vi "Read Ship States.vi"(11 "TCP Refnum In":refnum<k5>) -> (2 "Eta_ship":dbl[](array[numeric]), 3 "TCP Refnum Out":refnum<k5>)   [LabVIEW 2014]
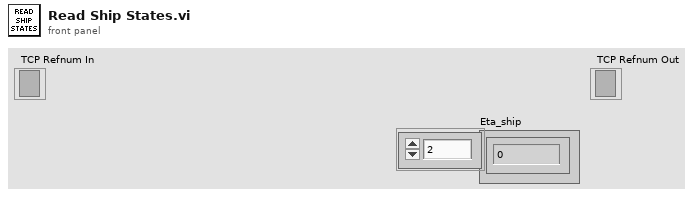
[diagram p1: front panel]
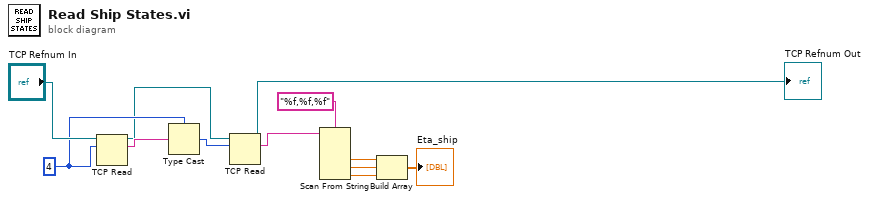
[diagram p0: block diagram]
diagram:
  w10 = 4
  n1 = TCP Read(connection ID="TCP Refnum In", bytes to read=w10) -> (connection ID out=w8:refnum<k5>, data out=w11:string)  [unwired: 3 in, 1 out]
  n2 = Type Cast(type=w10, x=w11) -> (*(type *) &x=w9:i32)
  n3 = TCP Read(connection ID=w8, bytes to read=w9) -> (connection ID out=→"TCP Refnum Out":refnum<k5>, data out=w6:string)  [unwired: 3 in, 1 out]
  n4 = Scan From String(format string="%f,%f,%f", input string=w6) -> (output 1=w4:dbl, output 2=w3:dbl, output 3=w2:dbl)  [unwired: 5 in, 3 out]
  n5 = Build Array(w4, w3, w2) -> (→"Eta_ship":dbl[])
